vi "Engine Init Test.vi"() -> ()   [LabVIEW 2020]
uses:
  Engine/Get Engine Ref.vi
  Engine/Engine.lvclass
panel:
  out "Same Ref?":bool
  out "VersionString 2":string
  out "error out":errorcluster
  out "VersionString":string
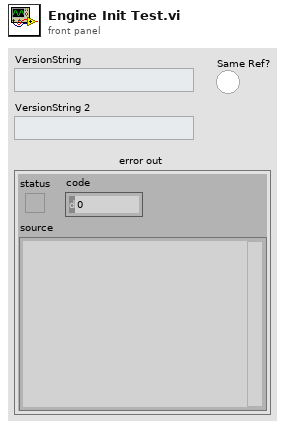
[diagram p1: front panel]
types:
  T1 = typedef "TSS.lvlib/Engine.lvclass/Session Handle.ctl" = refnum<data-value>
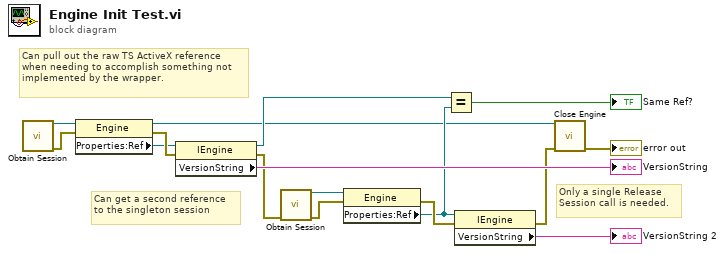
[diagram p0: block diagram]
diagram:
  # "Can pull out the raw TS ActiveX reference when needing to accomplish something not implemented by the wrapper."
  # "Only a single Release Session call is needed."
  # "Can get a second reference to the singleton session"
  n1 = call "Obtain Session.vi"() -> ("Session Handle"=w10:T1, "error out"=w9:errorcluster)  [unwired: 14 in]
  n2 = property class="Engine"(reference=w10, error in=w9) -> (reference out=w1:T1, error out=w15:errorcluster, "Properties:Ref"=w4:refnum<k7>)
  n3 = property class="IEngine"(reference=w4, error in=w15) -> (reference out=w12:refnum<k7>, error out=w8:errorcluster, "VersionString"=→"VersionString":string)
  n4 = call "Obtain Session.vi"("error in (no error)"=w8) -> ("Session Handle"=w7:T1, "error out"=w6:errorcluster)  [unwired: 13 in]
  n5 = property class="Engine"(reference=w7, error in=w6) -> (error out=w14:errorcluster, "Properties:Ref"=w5:refnum<k7>)  [unwired: 1 out]
  n6 = Equal?(x=w12, y=w5) -> (x = y?=→"Same Ref?":bool)
  n7 = property class="IEngine"(reference=w5, error in=w14) -> (error out=w2:errorcluster, "VersionString"=→"VersionString 2":string)  [unwired: 1 out]
  n8 = call "Close Engine.vi"("Session Handle in"=w1, "error in (no error)"=w2) -> ("error out"=→"error out":errorcluster)  [unwired: 13 in]
